vi "Camera.Simulated.RefToDVR.vi"(10 "Ref":u32 format="%08x") -> (2 "Ref":T1)   [LabVIEW 2013, in "Camera.Simulated.lvclass"]
uses:
  Camera.Simulated.lvclass
  Dependencies--Cluster.ctl
  PrivateData--Cluster.ctl
  PrivateData--Ref.ctl
  Configuration--CLuster.ctl
  CircularBuffer.ImageData/CircularBuffer.ImageData.lvclass
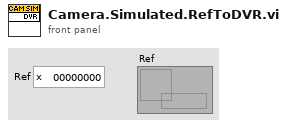
[diagram p1: front panel]
types:
  T1 = typedef "Camera.Simulated.lvclass/PrivateData--Ref.ctl" = refnum<data-value>
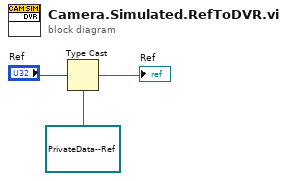
[diagram p0: block diagram]
diagram:
  n1 = Type Cast(type=T1 refnum ("Ref"), x="Ref") -> (*(type *) &x=→"Ref":T1)
